vi "Reference Enqueue Message (Single).vi"(6 "Priority Message? (F)":bool, 7 "VI Ref":refnum<vi>, 8 "error in":errorcluster, 9 "Message Data":variant, 10 "Message":string, 11 "Queue":string) -> (0 "error out":errorcluster, 3 "dup Message Queue":refnum<queue>)   [LabVIEW 2021, in "Message Queue.lvlib"]
doc: "Obtains a Reference to the Queue and enqueues the messaage. \nFor a regular message, enqueue the message. For a priority message, enqueue it at the front of the queue."
uses:
  Message Queue.lvlib
  Message Cluster.ctl
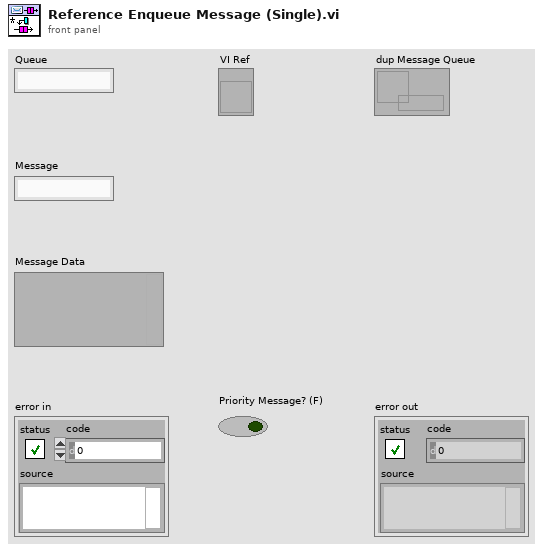
[diagram p1: front panel]
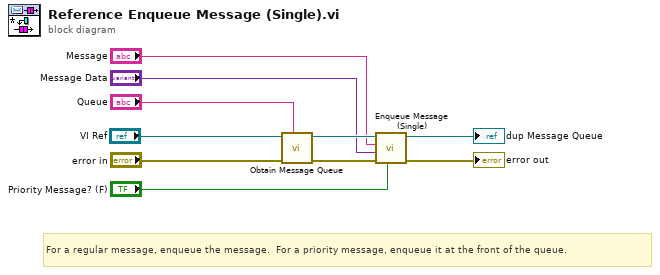
[diagram p0: block diagram]
diagram:
  # "For a regular message, enqueue the message.  For a priority message, enqueue it at the front of the queue."
  n1 = call "Obtain Message Queue.vi"("Queue"="Queue", "error in"="error in", "VI Ref"="VI Ref") -> ("error out"=w9:errorcluster, "Message Queue"=w7:refnum<queue>)  [unwired: 7 in]
  n2 = call "Enqueue Message (Single).vi"("Priority Message? (F)"="Priority Message? (F)", "error in (no error)"=w9, "Message Data"="Message Data", "Message"="Message", "Message Queue"=w7) -> ("error out"=→"error out":errorcluster, "dup Message Queue"=→"dup Message Queue":refnum<queue>)  [unwired: 5 in]
